vi "LJM_eReadAddress.vi"(0 "Handle In":i32, 5 "Address":i32, 7 "Type":i32, 11 "error in":errorcluster) -> (4 "Handle Out":i32, 10 "Value":dbl format="%.2f", 15 "error out":errorcluster)   [LabVIEW 2026]
uses:
  labjackm.dll
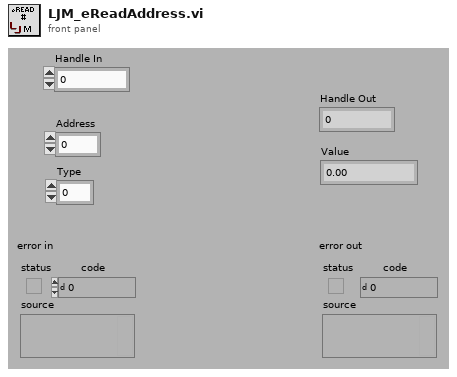
[diagram p1: front panel]
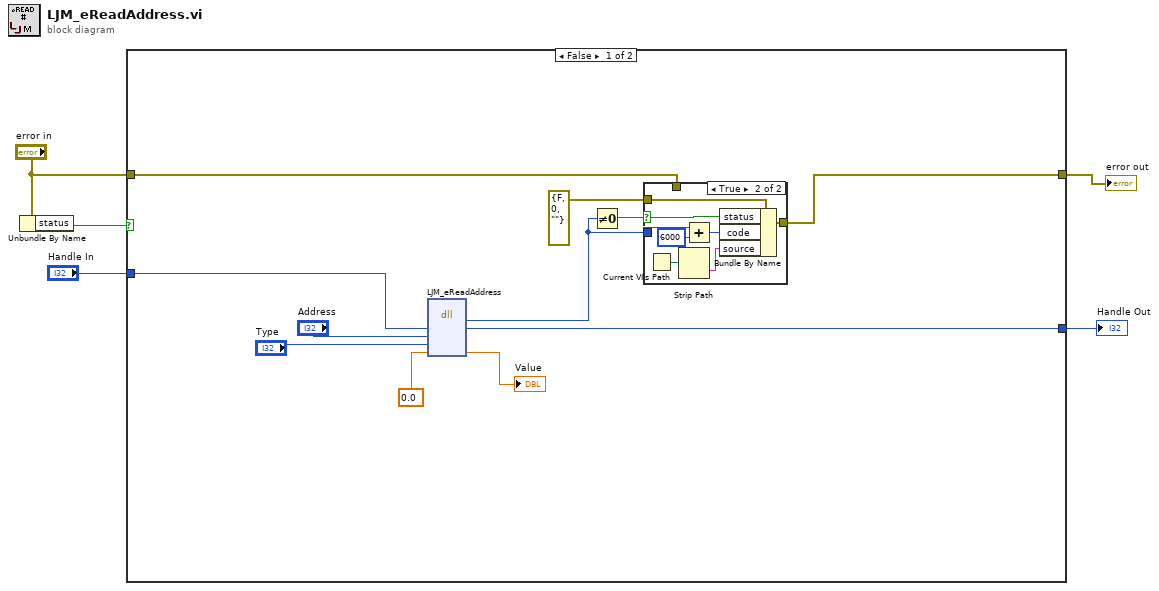
[diagram p0: block diagram]
diagram:
  n1 = Unbundle By Name("error in") -> ("status"=w5:bool)
  n2 = case shown="False" w5 {
    tunnel: "error in" -> [w13 w27]
    tunnel: [w12 w27] -> w3
    tunnel: "Handle In" -> [w7 w26]
    tunnel: [w6 w26] -> w1
    frame False {
      n3 = dll-call lib="labjackm.dll" fn="LJM_eReadAddress"("Handle"=w7, "Address"="Address", "Type"="Type", "Value"=0.0 ("ErrorFrame")) -> (w16:i32, "Handle"=w6:i32, "Value"=→"Value":dbl)  [unwired: 5 in, 2 out]
      n4 = Not Equal To 0?(x=w16) -> (x != 0?=w15:bool)
      n5 = case shown="True" w15 {
        selector: w15 -> [_ w24]
        tunnel: [w17 w25] -> w12
        tunnel: errorcluster {"status"=FALSE, "code"=0, "source"=""} ("error IO") -> [_ w23]
        tunnel: w16 -> [_ w19]
        tunnel: w13 -> [w17 _]
        frame False {
        }
        frame True {
          n6 = Current VI's Path() -> (path=w21:path)
          n7 = Strip Path(path=w21) -> (name=w22:string)  [unwired: 1 out]
          n8 = Add(x=w19, y=6000) -> (x+y=w20:i32)
          n9 = Bundle By Name(cluster=w23, "status"=w24, "code"=w20, "source"=w22) -> (w25:errorcluster)
        }
      }
    }
    frame True {
    }
  }
  "error out" <- w3
  "Handle Out" <- w1
